vi "tm485_lightsheet.vi"() -> ()   [LabVIEW 2023, in "HamamatsuCam.lvlib" / "HamamatsuCam.lvclass"]
uses:
  HamamatsuCam/HamamatsuCam/HamamatsuCam.lvclass
panel:
  in  "Internal Line Interval":dbl=9.74436e-06
  in  "Readout Direction":u32(ring)=1 items=["FORWARD"=1, "BACKWARD"=2]
  in  "Pre Hsync Count":u32
  out "Image":u16[][](graph)
  out "Frames Per Second":dbl
  in  "Quit":bool
  out "Error Out":errorcluster {"code" format="%.0x"}
  # "This is just a simple example\nof how to setup a camera for\na Lightsheet application with\na Flash4.0 V2"
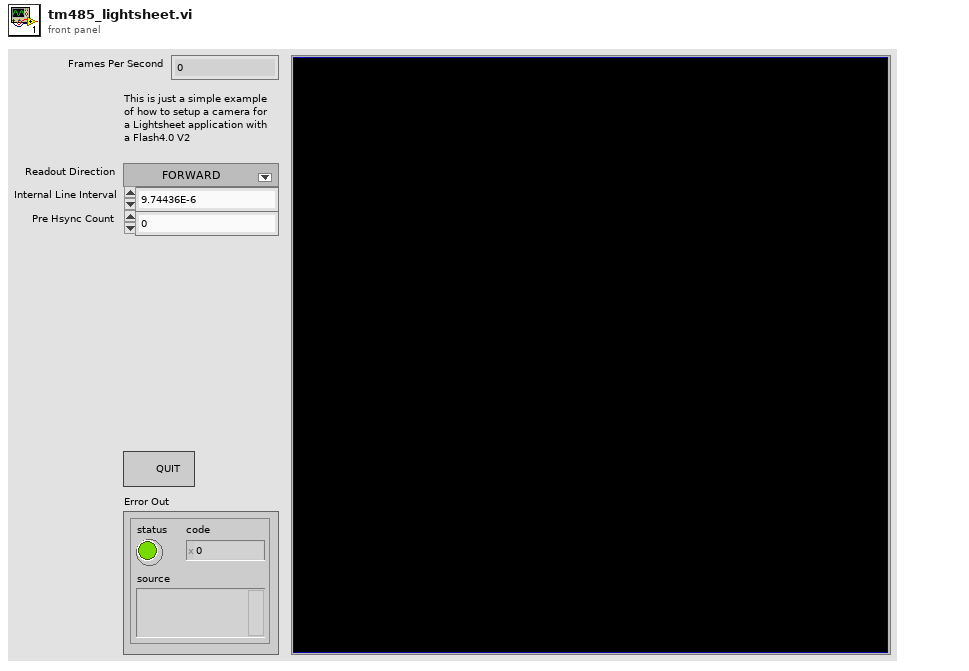
[diagram p1: front panel]
types:
  T1 = cluster{"Output Trigger Mode":u32, "Output Trigger Polarity":u32}
  T2 = cluster{"Output Trigger Period":dbl, "Delay":dbl, "Source":u32}
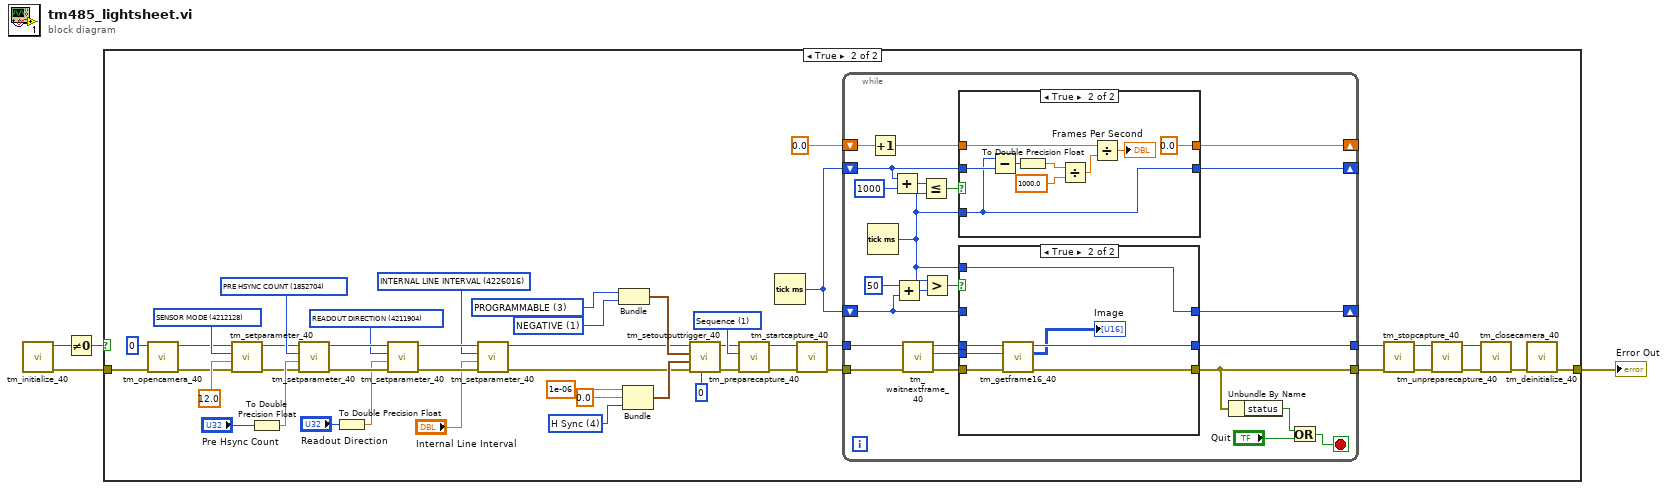
[diagram p0: block diagram]
diagram:
  n1 = call "tm_initialize_40.vi"() -> ("error out"=w1:errorcluster, "Number Of Cameras"=w2:u32)  [unwired: 8 in, 2 out]
  n2 = Not Equal To 0?(x=w2) -> (x != 0?=w4:bool)
  n3 = case shown="True" w4 {
    tunnel: w1 -> [w5 w52]
    tunnel: [w5 w49] -> w3
    frame False {
    }
    frame True {
      w20 = u32 1 items=["NEGATIVE"=1, "POSITIVE"=2] ("Output Trigger Polarity")
      w12 = u32 3 items=["LOW"=1, "GLOBAL EXPOSURE"=2, "PROGRAMMABLE"=3, "TRIGGER READY"=4, "HIGH"=5] ("Output Trigger Mode")
      w15 = u32 4 items=["Exposure"=1, "Readout End"=2, "V Sync"=3, "H Sync"=4, "Trigger"=6] ("Source")
      w21 = u32 4226016 items=["SENSOR MODE"=4212128, "CCD MODE"=4212384, "READOUT MODE"=4211872, "ACTIVE VIEW INDEX"=4343136, "BITS PER CHANNEL"=4342976, "IMAGE PIXEL TYPE"=4343296, "BINNING"=4215968, "EXPOSURE TIME"=2049184, "CONTRAST GAIN"=3163312, "CONTRAST OFFSET"=3163328, "LIGHT MODE"=2114720, "SENSITIVITY"=2114992, "PHOTON IMAGING MODE"=2115200, "HIGH DYNAMIC RANGE MODE"=3163360, "WHITE BALANCE"=3163568, "TEMPERATURE"=2115232, "TEMPERATURE TARGET"=2115264, "SENSOR COOLER FAN"=2115296, "LINEBUNDLE HEIGHT"=4212192, "MECHANICAL SHUTTER"=2115488, "BACK FOCUS POSITION"=8422304, "TRIGGER CONNECTOR"=1066432, "TRIGGER SOURCE"=1066144, "OUTPUT TRIGGER SOURCE"=1852576, "TRIGGER GLOBAL EXPOSURE"=2049680, "FIRST TRIGGER BEHAVIOR"=2049696, "CHANNEL SYNC"=1852352, "READOUT DIRECTION"=4211904, "PRE HSYNC COUNT"=1852704, "INTERNAL LINE SPEED"=4226000, "INTERNAL LINE INTERVAL"=4226016] ("Parameter")
      w25 = u32 4212128 items=["SENSOR MODE"=4212128, "CCD MODE"=4212384, "READOUT MODE"=4211872, "ACTIVE VIEW INDEX"=4343136, "BITS PER CHANNEL"=4342976, "IMAGE PIXEL TYPE"=4343296, "BINNING"=4215968, "EXPOSURE TIME"=2049184, "CONTRAST GAIN"=3163312, "CONTRAST OFFSET"=3163328, "LIGHT MODE"=2114720, "SENSITIVITY"=2114992, "PHOTON IMAGING MODE"=2115200, "HIGH DYNAMIC RANGE MODE"=3163360, "WHITE BALANCE"=3163568, "TEMPERATURE"=2115232, "TEMPERATURE TARGET"=2115264, "SENSOR COOLER FAN"=2115296, "LINEBUNDLE HEIGHT"=4212192, "MECHANICAL SHUTTER"=2115488, "BACK FOCUS POSITION"=8422304, "TRIGGER CONNECTOR"=1066432, "TRIGGER SOURCE"=1066144, "OUTPUT TRIGGER SOURCE"=1852576, "TRIGGER GLOBAL EXPOSURE"=2049680, "FIRST TRIGGER BEHAVIOR"=2049696, "CHANNEL SYNC"=1852352, "READOUT DIRECTION"=4211904, "PRE HSYNC COUNT"=1852704, "INTERNAL LINE SPEED"=4191408, "INTERNAL LINE INTERVAL"=4191424] ("Parameter")
      w26 = u32 1852704 items=["SENSOR MODE"=4212128, "CCD MODE"=4212384, "READOUT MODE"=4211872, "ACTIVE VIEW INDEX"=4343136, "BITS PER CHANNEL"=4342976, "IMAGE PIXEL TYPE"=4343296, "BINNING"=4215968, "EXPOSURE TIME"=2049184, "CONTRAST GAIN"=3163312, "CONTRAST OFFSET"=3163328, "LIGHT MODE"=2114720, "SENSITIVITY"=2114992, "PHOTON IMAGING MODE"=2115200, "HIGH DYNAMIC RANGE MODE"=3163360, "WHITE BALANCE"=3163568, "TEMPERATURE"=2115232, "TEMPERATURE TARGET"=2115264, "SENSOR COOLER FAN"=2115296, "LINEBUNDLE HEIGHT"=4212192, "MECHANICAL SHUTTER"=2115488, "BACK FOCUS POSITION"=8422304, "TRIGGER CONNECTOR"=1066432, "TRIGGER SOURCE"=1066144, "OUTPUT TRIGGER SOURCE"=1852576, "TRIGGER GLOBAL EXPOSURE"=2049680, "FIRST TRIGGER BEHAVIOR"=2049696, "CHANNEL SYNC"=1852352, "READOUT DIRECTION"=4211904, "PRE HSYNC COUNT"=1852704, "INTERNAL LINE SPEED"=4191408, "INTERNAL LINE INTERVAL"=4191424] ("Parameter")
      w27 = u32 4211904 items=["SENSOR MODE"=4212128, "CCD MODE"=4212384, "READOUT MODE"=4211872, "ACTIVE VIEW INDEX"=4343136, "BITS PER CHANNEL"=4342976, "IMAGE PIXEL TYPE"=4343296, "BINNING"=4215968, "EXPOSURE TIME"=2049184, "CONTRAST GAIN"=3163312, "CONTRAST OFFSET"=3163328, "LIGHT MODE"=2114720, "SENSITIVITY"=2114992, "PHOTON IMAGING MODE"=2115200, "HIGH DYNAMIC RANGE MODE"=3163360, "WHITE BALANCE"=3163568, "TEMPERATURE"=2115232, "TEMPERATURE TARGET"=2115264, "SENSOR COOLER FAN"=2115296, "LINEBUNDLE HEIGHT"=4212192, "MECHANICAL SHUTTER"=2115488, "BACK FOCUS POSITION"=8422304, "TRIGGER CONNECTOR"=1066432, "TRIGGER SOURCE"=1066144, "OUTPUT TRIGGER SOURCE"=1852576, "TRIGGER GLOBAL EXPOSURE"=2049680, "FIRST TRIGGER BEHAVIOR"=2049696, "CHANNEL SYNC"=1852352, "READOUT DIRECTION"=4211904, "PRE HSYNC COUNT"=1852704, "INTERNAL LINE SPEED"=4191408, "INTERNAL LINE INTERVAL"=4191424] ("Parameter")
      w40 = 1 items=["Snap", "Sequence"] ("Capture mode")
      n4 = call "tm_opencamera_40.vi"("error in (no error)"=w52, "Camera Index"=u32 0) -> ("error out"=w11:errorcluster, "Handle out"=w10:u32)  [unwired: 7 in, 1 out]
      n5 = call "tm_setparameter_40.vi"("error in (no error)"=w11, "Value in"=12.0, "Parameter"=w25, "Handle in"=w10) -> ("error out"=w13:errorcluster, "Handle out"=w14:u32)  [unwired: 6 in]
      n6 = To Double Precision Float(number="Pre Hsync Count") -> (double precision float=w34:dbl)
      n7 = call "tm_setparameter_40.vi"("error in (no error)"=w13, "Value in"=w34, "Parameter"=w26, "Handle in"=w14) -> ("error out"=w32:errorcluster, "Handle out"=w31:u32)  [unwired: 6 in]
      n8 = To Double Precision Float(number="Readout Direction") -> (double precision float=w30:dbl)
      n9 = call "tm_setparameter_40.vi"("error in (no error)"=w32, "Value in"=w30, "Parameter"=w27, "Handle in"=w31) -> ("error out"=w23:errorcluster, "Handle out"=w24:u32)  [unwired: 6 in]
      n10 = call "tm_setparameter_40.vi"("error in (no error)"=w23, "Value in"="Internal Line Interval", "Parameter"=w21, "Handle in"=w24) -> ("error out"=w6:errorcluster, "Handle out"=w7:u32)  [unwired: 6 in]
      n11 = Bundle("Output Trigger Mode"=w12, "Output Trigger Polarity"=w20) -> (w19:T1)  [unwired: 1 in]
      n12 = Bundle("Output Trigger Period"=1e-06, "Delay"=0.0, "Source"=w15) -> (w18:T2)  [unwired: 1 in]
      n13 = call "tm_setoutputtrigger_40.vi"("Port"=0 ("Index"), "error in (no error)"=w6, "Programmable Options"=w18, "Type"=w19, "Handle in"=w7) -> ("error out"=w9:errorcluster, "Handle out"=w8:u32)  [unwired: 5 in]
      n14 = call "tm_preparecapture_40.vi"("error in (no error)"=w9, "Capture mode"=w40, "Handle in"=w8) -> ("error out"=w38:errorcluster, "Handle out"=w39:u32)  [unwired: 5 in, 2 out]
      n15 = Tick Count (ms)() -> (millisecond timer value=w36:u32)
      n16 = call "tm_startcapture_40.vi"("error in (no error)"=w38, "Handle in"=w39) -> ("error out"=w41:errorcluster, "Handle out"=w42:u32)  [unwired: 8 in]
      n17 = while {
        tunnel: [w55] -> w45
        tunnel: [w56] -> w46
        tunnel: w42 -> [w73]
        tunnel: w41 -> [w74]
        shift-right: [w71] -> _
        shift-left: w36 -> [w68]
        shift-right: [w72] -> _
        shift-left: 0.0 -> [w65]
        shift-right: [w54] -> _
        shift-left: w36 -> [w57]
        stop <- w53 stop-if-true
        n18 = Tick Count (ms)() -> (millisecond timer value=w58:u32)
        n19 = Increment(x=w65) -> (x+1=w66:dbl)
        n20 = Add(x=w68, y=u32 1000) -> (x+y=w70:u32)
        n21 = Add(x=u32 50, y=w57) -> (x+y=w60:u32)
        n22 = call "tm_waitnextframe_40.vi"("error in (no error)"=w74, "Handle in"=w73) -> ("error out"=w63:errorcluster, "Frame Index"=w62:i32, "Handle out"=w64:u32)  [unwired: 6 in, 1 out]
        n23 = Less Or Equal?(x=w70, y=w58) -> (x <= y?=w67:bool)
        n24 = Greater?(x=w58, y=w60) -> (0:w59:bool)
        n25 = case shown="True" w67 {
          tunnel: w68 -> [w88 w91]
          tunnel: [w88 w89] -> w71
          tunnel: w66 -> [w87 w95]
          tunnel: w58 -> [_ w89]
          tunnel: [w87 0.0] -> w72
          frame False {
          }
          frame True {
            n26 = Subtract(x=w89, y=w91) -> (x-y=w90:u32)
            n27 = To Double Precision Float(number=w90) -> (double precision float=w97:dbl)
            n28 = Divide(x=w97, y=1000.0) -> (x/y=w94:dbl)
            n29 = Divide(x=w95, y=w94) -> (x/y=→"Frames Per Second":dbl)
          }
        }
        n30 = case shown="True" w59 {
          tunnel: w64 -> [w79 w86]
          tunnel: w63 -> [w78 w85]
          tunnel: w62 -> [_ w84]
          tunnel: w57 -> [w77 _]
          tunnel: w58 -> [_ w83]
          tunnel: [w79 w81] -> w55
          tunnel: [w78 w82] -> w56
          tunnel: [w77 w83] -> w54
          frame False {
          }
          frame True {
            n31 = call "tm_getframe16_40.vi"("error in (no error)"=w85, "Frame Index"=w84, "Handle in"=w86) -> ("error out"=w82:errorcluster, "Data"=→"Image":u16[][], "Handle out"=w81:u32)  [unwired: 5 in, 1 out]
          }
        }
        n32 = Unbundle By Name(w56) -> ("status"=w76:bool)
        n33 = Or(x=w76, y="Quit") -> (x .or. y?=w53:bool)
      }
      n34 = call "tm_stopcapture_40.vi"("error in (no error)"=w46, "Handle in"=w45) -> ("error out"=w43:errorcluster, "Handle out"=w44:u32)  [unwired: 8 in]
      n35 = call "tm_unpreparecapture_40.vi"("error in (no error)"=w43, "Handle in"=w44) -> ("error out"=w48:errorcluster, "Handle out"=w47:u32)  [unwired: 8 in]
      n36 = call "tm_closecamera_40.vi"("error in (no error)"=w48, "Handle in"=w47) -> ("error out"=w50:errorcluster)  [unwired: 9 in]
      n37 = call "tm_deinitialize_40.vi"("error in (no error)"=w50) -> ("error out"=w49:errorcluster)  [unwired: 10 in]
    }
  }
  "Error Out" <- w3
